vi "XY Graph Denoise Plot.vi"(7 "Wavelet Analysis Options":T4={"Wavelet"=enum."db02", "Option for Approximate Coefficients"=enum."None", "# Levels"=1, "Threshold Settings"={"Thresholding Rule"=enum."Universal", "Rescaling Method"=enum."Single level", "Soft Threshold?"=TRUE}, "Wavelet Transform Type"=enum."Discrete"}, 8 "error in (no error)":errorcluster, 9 "Replace Plot (T)?":bool=TRUE, 11 "Selected Plot Info":T1={"Multiplot XY Graph"=refnum, "Mouse Coordinates"={"Horizontal"=0, "Vertical"=0}, "Plot Index"=-1}) -> (0 "Error Out":errorcluster, 1 "Message":string, 3 "Denoised Plot":cluster{"t Array":dbl[], "IRF Array":dbl[]})   [LabVIEW 2021, in "XY Graph Add-Ons.lvlib"]
uses:
  XY Graph Add-Ons.lvlib
  Math/Advanced Signal Processing Toolkit/Wavelet Analysis Options.ctl
  XY Graph Selected Plot Info.ctl
  XY Graph Refnum.ctl
  <vilib>/Utility/miscctls.llb/LVPoint32TypeDef.ctl
  <vilib>/addons/Wavelet Analysis/application.llb/WA Denoise (DWT Real Array).vi
  <vilib>/addons/Wavelet Analysis/application.llb/WA Denoise (UWT Real Array).vi
  <vilib>/addons/_Advanced Signal Processing/NI_AdvSigProcWA.lvlib
  Math/Math.lvlib
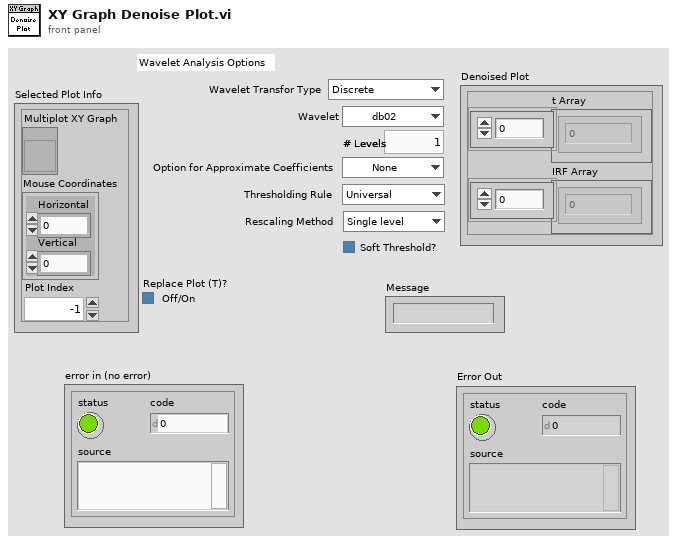
[diagram p1: front panel]
types:
  T1 = typedef "XY Graph Add-Ons.lvlib/XY Graph Selected Plot Info.ctl" = cluster{"Multiplot XY Graph":T2, "Mouse Coordinates":T3, "Plot Index":i32}
  T2 = typedef "XY Graph Add-Ons.lvlib/XY Graph Refnum.ctl" = refnum<vi>
  T3 = typedef "LVPoint32TypeDef.ctl" = cluster{"Horizontal":i32, "Vertical":i32}
  T4 = typedef "Math.lvlib/Wavelet Analysis Options.ctl" = cluster{"Wavelet":enum16{"db02", "db03", "db04", "db05", "db06", "db07", "db08", "db09", "db10", "db11", "db12", "db13", "db14", "Haar", "bior1_3", "bior1_5", "bior2_2", "bior2_4", "bior2_6", "bior2_8", "bior3_1", "bior3_3", "bior3_5", "bior3_7", "bior3_9", "bior4_4 (FBI)", "bior5_5", "bior6_8", "coif1", "coif2", "coif3", "coif4", "coif5", "sym2", "sym3", "sym4", "sym5", "sym6", "sym7", "sym8"}, "Option for Approximate Coefficients":enum16{"None", "Threshold", "Detrend"}, "# Levels":i32, "Threshold Settings":cluster{"Thresholding Rule":enum16{"SURE", "Hybrid", "Universal", "Minimax"}, "Rescaling Method":enum16{"One", "Single level", "Multiple levels"}, "Soft Threshold?":bool}, "Wavelet Transform Type":enum16{"Discrete", "Undecimated"}}
  T5 = cluster{"Thresholding Rule":enum16{"SURE", "Hybrid", "Universal", "Minimax"}, "Rescaling Method":enum16{"One", "Single level", "Multiple levels"}, "Soft Threshold?":bool}
  T6 = enum16{"db02", "db03", "db04", "db05", "db06", "db07", "db08", "db09", "db10", "db11", "db12", "db13", "db14", "Haar", "bior1_3", "bior1_5", "bior2_2", "bior2_4", "bior2_6", "bior2_8", "bior3_1", "bior3_3", "bior3_5", "bior3_7", "bior3_9", "bior4_4 (FBI)", "bior5_5", "bior6_8", "coif1", "coif2", "coif3", "coif4", "coif5", "sym2", "sym3", "sym4", "sym5", "sym6", "sym7", "sym8"}
  T7 = cluster{"X Array":dbl[], "denoised signal":dbl[]}
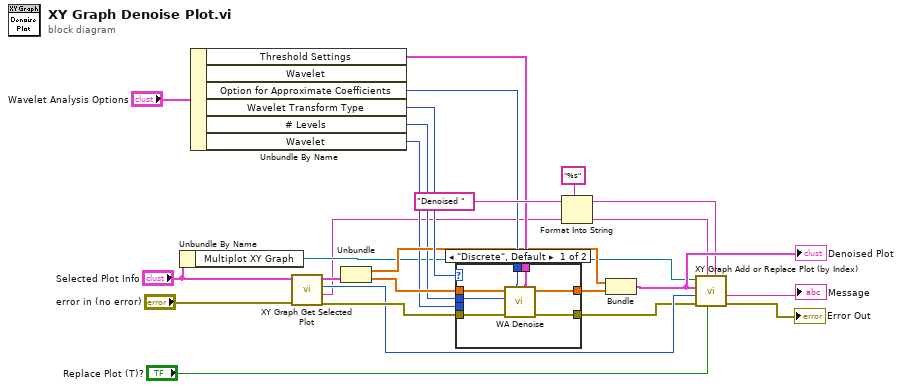
[diagram p0: block diagram]
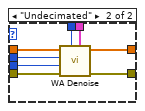
[diagram p2: hidden frame]
diagram:
  n1 = Unbundle By Name("Selected Plot Info") -> ("Multiplot XY Graph"=w8:T2)
  n2 = Unbundle By Name("Wavelet Analysis Options") -> ("Threshold Settings"=w17:T5, "Option for Approximate Coefficients"=w18:enum16{"None", "Threshold", "Detrend"}, "Wavelet Transform Type"=w16:enum16{"Discrete", "Undecimated"}, "# Levels"=w10:i32, "Wavelet"=w11:T6)  [unwired: 1 out]
  n3 = call "XY Graph Get Selected Plot.vi"("error in (no error)"="error in (no error)", "Selected Plot Info"="Selected Plot Info") -> ("error out"=w20:errorcluster, "Plot Name"=w5:string, "Plot Index"=w7:i32, "Plot"=w14:cluster{"X Array":dbl[], "Y Array":dbl[]})  [unwired: 4 in, 2 out]
  n4 = Unbundle(w14) -> ("X Array"=w12:dbl[], "Y Array"=w13:dbl[])
  n5 = case shown="\"Discrete\", Default" w16 {
    tunnel: w13 -> [w31 w39]
    tunnel: [w27 w38] -> w21
    tunnel: w20 -> [w29 w37]
    tunnel: [w28 w36] -> w6
    tunnel: w11 -> [_ w35]
    tunnel: w18 -> [w26 w34]
    tunnel: w10 -> [w30 w33]
    tunnel: w17 -> [w25 w32]
    frame "Discrete", Default {
      n6 = call-poly <vilib>:"WA Denoise.vi"("threshold settings"=w25, "option for approx coef"=w26, "error in (no error)"=w29, "levels"=w30, "signal"=w31) -> ("error out"=w28:errorcluster, "denoised signal"=w27:dbl[])  [unwired: 5 in]
    }
    frame "Undecimated" {
      n7 = call-poly <vilib>:"WA Denoise.vi"("threshold settings"=w32, "option for approx coef"=w34, "error in (no error)"=w37, "wavelet"=w35, "levels"=w33, "signal"=w39) -> ("error out"=w36:errorcluster, "denoised signal"=w38:dbl[])  [unwired: 4 in]
    }
  }
  n8 = Format Into String(format string="%s", initial string="Denoised ", w5) -> (resulting string=w4:string)  [unwired: 1 in, 1 out]
  n9 = Bundle("X Array"=w12, "denoised signal"=w21) -> (w9:T7)  [unwired: 1 in]
  "Denoised Plot" <- w9
  n10 = call "XY Graph Add or Replace Plot (by Index).vi"("New Plot Name"=w4, "Replace Plot (T)?"="Replace Plot (T)?", "Original Plot Name"=w5, "error in (no error)"=w6, "Plot Index"=w7, "Plot in"=w9, "XYGraph in"=w8) -> ("error out"=→"Error Out":errorcluster, "Message"=→"Message":string)  [unwired: 3 in]
